vi "Invalid Handle Error Code.vi"() -> (0 "Invalid Handle Error":i32)   [LabVIEW 2024, in "serenial.io-ase.test.lvlib"]
uses:
  serenial.io-ase.test.lvlib
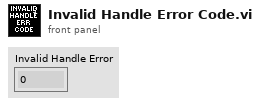
[diagram p1: front panel]
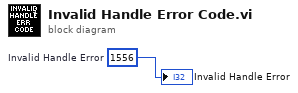
[diagram p0: block diagram]
diagram:
  w1 = 1556  # Invalid Handle Error
  "Invalid Handle Error" <- w1
